vi "Init WebView2 Core.vi"(8 "error in (no error)":errorcluster, 11 "WebView in":refnum<class "WebView.lvclass">) -> (0 "error out":errorcluster, 3 "WebView out":refnum<class "WebView.lvclass">)   [LabVIEW 2020, in "WebView.lvclass"]
uses:
  WebView.lvclass
  WebView.lvclass/WebView.ctl
  <vilib>/sklein/WebView2/Libs/Microsoft.Web.WebView2.WinForms.dll
  <vilib>/sklein/WebView2/Libs/Microsoft.Web.WebView2.Core.dll
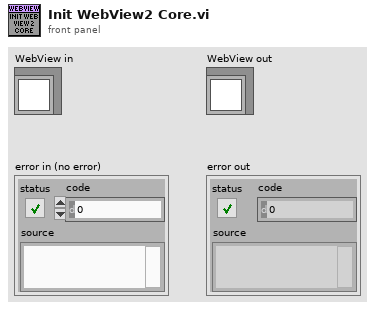
[diagram p1: front panel]
types:
  T1 = typedef "WebView.lvclass/Resources--cluster.ctl" = cluster{"WebView2 Control":refnum<k24>, "Webview2 Core":refnum<k24>, "event callback":refnum<k27>, "Environment":refnum<k24>}
  T2 = typedef "WebView.lvclass/Paths-cluster.ctl" = cluster{"Webview2 Native":path, "Edge Application":path, "User Data":path}
  T3 = typedef "WebView.lvclass/Core Envrionment Options--cluster.ctl" = cluster{"additionalBrowserArguments":string, "language":string, "targetCompatibleBrowserVersion":string, "allowSingleSignOnUsingOSPrimaryAccount":bool}
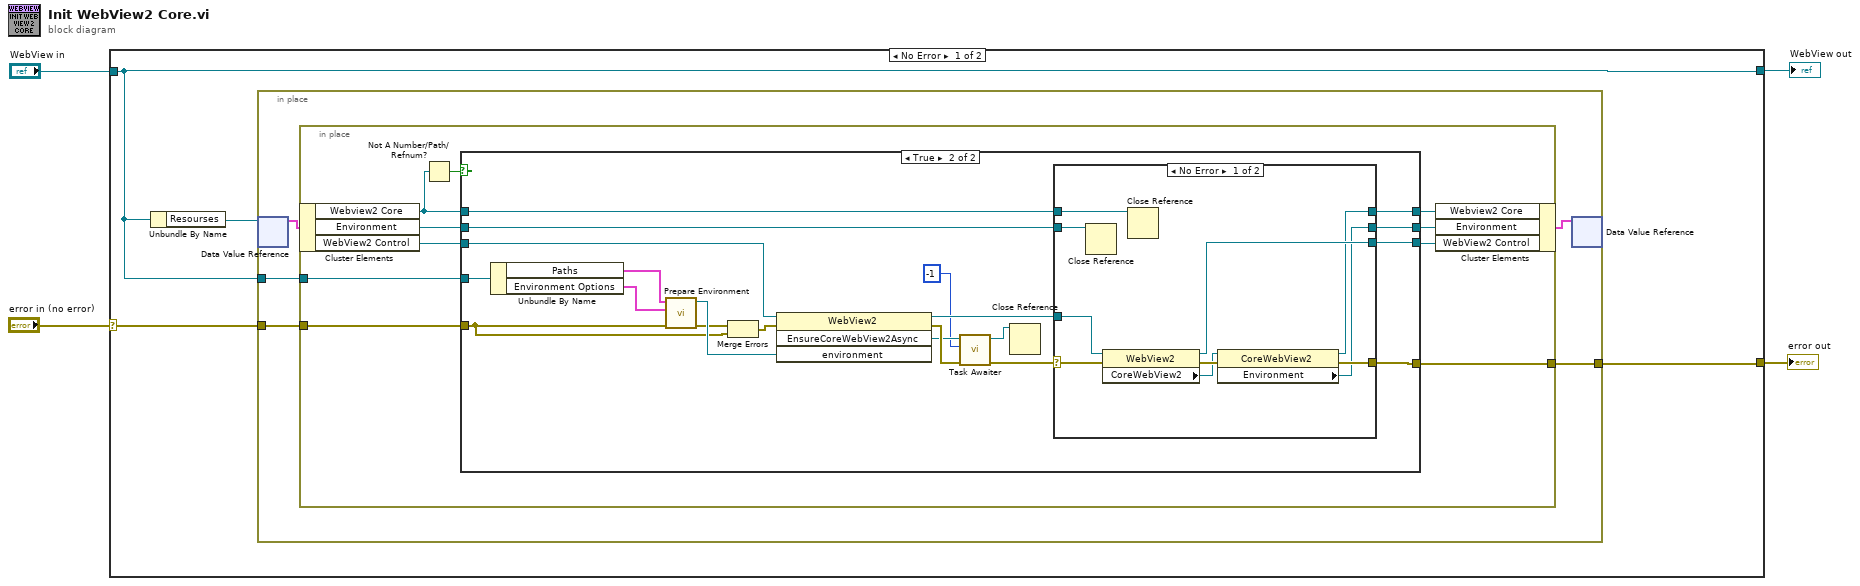
[diagram p0: block diagram]
diagram:
  n1 = case shown="No Error" "error in (no error)" {
    selector: "error in (no error)" -> [w7 w63]
    tunnel: [w8 w63] -> w4
    tunnel: [w6 w62] -> w1
    tunnel: "WebView in" -> [w6 w62]
    frame No Error {
      n2 = Unbundle By Name(w6) -> ("Resourses"=w5:refnum<data-value>)
      n3 = in-place {
        in-place-border: [w13] -> w8
        in-place-border: w6 -> [w12]
        in-place-border: w7 -> [w11]
        n4 = in-place-dvr #1(w5) -> (w10:T1)  [unwired: 1 out]
        n5 = in-place {
          in-place-border: [w22] -> w13
          in-place-border: w11 -> [w20]
          in-place-border: w12 -> [w18]
          n6 = in-place-cluster #2(w10) -> ("Webview2 Core"=w21:refnum<k24>, "Environment"=w16:refnum<k24>, "WebView2 Control"=w15:refnum<k24>)
          n7 = Not A Number/Path/Refnum?(number/path/refnum=w21) -> (NaN/Path/Refnum?=w23:bool)
          n8 = case shown="True" w23 {
            tunnel: [w27 w43] -> w19
            tunnel: w21 -> [w27 w42]
            tunnel: w20 -> [w26 w28]
            tunnel: [w26 w44] -> w22
            tunnel: [w24 w46] -> w14
            tunnel: w18 -> [_ w45]
            tunnel: [w25 w41] -> w17
            tunnel: w16 -> [w25 w40]
            tunnel: w15 -> [w24 w31]
            frame False {
            }
            frame True {
              n9 = Unbundle By Name(w45) -> ("Paths"=w29:T2, "Environment Options"=w39:T3)
              n10 = call "Prepare Environment.vi"("error in"=w28, "Envrionment Options"=w39, "Paths"=w29) -> ("error out"=w32:errorcluster, "Environment out"=w38:refnum<k24>)  [unwired: 7 in]
              n11 = Merge Errors(w32, w28) -> (w30:errorcluster)
              n12 = invoke class="WebView2" method="EnsureCoreWebView2Async"(reference=w31, error in=w30, "environment"=w38) -> (reference out=w47:refnum<k24>, error out=w37:errorcluster, "EnsureCoreWebView2Async"=w34:refnum<k24>)  [unwired: 1 in, 1 out]
              n13 = call "Task Awaiter.vi"("error in (no error)"=w37, "Timeout"=-1, "Task"=w34) -> ("error out"=w36:errorcluster, "Task"=w35:refnum<k24>)  [unwired: 6 in, 1 out]
              n14 = Close Reference(reference=w35) -> ()  [unwired: 1 in, 1 out]
              n15 = case shown="No Error" w36 {
                selector: w36 -> [w55 w59]
                tunnel: w47 -> [w57 w60]
                tunnel: [w50 w61] -> w43
                tunnel: [w56 w60] -> w46
                tunnel: [w52 w59] -> w44
                tunnel: w42 -> [w53 w61]
                tunnel: [w49 w58] -> w41
                tunnel: w40 -> [w48 w58]
                frame No Error {
                  n16 = Close Reference(reference=w48) -> ()  [unwired: 1 in, 1 out]
                  n17 = property class="WebView2"(reference=w57, error in=w55) -> (reference out=w56:refnum<k24>, error out=w54:errorcluster, "CoreWebView2"=w51:refnum<k24>)
                  n18 = Close Reference(reference=w53) -> ()  [unwired: 1 in, 1 out]
                  n19 = property class="CoreWebView2"(reference=w51, error in=w54) -> (reference out=w50:refnum<k24>, error out=w52:errorcluster, "Environment"=w49:refnum<k24>)
                }
                frame Error {
                }
              }
            }
          }
          n20 = in-place-cluster #2("Webview2 Core"=w19, "Environment"=w17, "WebView2 Control"=w14) -> (w9:T1)
        }
        n21 = in-place-dvr #1(w9) -> ()  [unwired: 2 out]
      }
    }
    frame Error {
    }
  }
  "error out" <- w4
  "WebView out" <- w1
